vi "PH_PowerUnit_BaseClass.handle TO.vi"(0 "VI in":refnum<vi>, 2 "String":string, 5 "error in (no error)":errorcluster) -> (14 "VI out":refnum<vi>, 19 "error out":errorcluster)   [LabVIEW 2014, in "PH_PowerUnit_BaseClass.lvlib"]
uses:
  PH_PowerUnit_BaseClass.lvlib
  PHELIX/PH_Sequencer/PH_Sequencer.lvlib
  PH_Common/PH_Common.lvlib
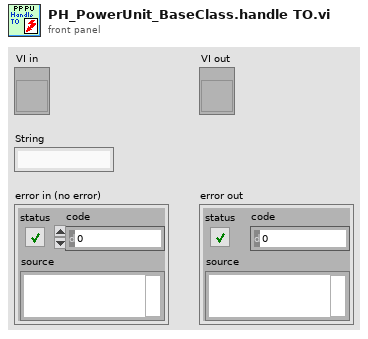
[diagram p1: front panel]
types:
  T1 = typedef "PH_PowerUnit_BaseClass.lvlib/PH_PowerUnit_BaseClass.i attribute.ctl" = cluster{"Constructor finished":bool, "PU":cluster{"In use":bool, "Service ID in use":i32, "GUI Ref":refnum<vi>}, "Enabling":cluster{"State":T2, "GUI Ref":refnum<vi>}, "Timing":cluster{"Last Shot":dbl, "Time between Shots [Sec]":dbl, "Waiting Time over?":bool, "Service ID Waiting Time":i32, "GUI Ref":refnum<vi>, "Instance":cluster{"Status":T3, "linked?":bool, "GUI Ref":refnum<vi>}}, "Sequencer":cluster{"SM State":string, "GUI Ref":refnum<vi>, "linked":bool}, "Subscribed Trendmssgs":cluster{"Tagname":string, "Status":T3, "linked?":bool, "Shot Condition":T3, "GUI Ref":refnum<vi>}[], "PP PU":T4, "Default Voltage (V)":dbl, "GUI Refs":T5, "PSDB data":cluster{"Shot Voltage [V]":dbl, "State TO SM":T6, "Write 2 early":bool}, "State TO SM":T6}
  T2 = typedef "PH_SystemInformation.lvlib/PH_SystemInformationEnabling State.ctl" = i32
  T3 = typedef "PH_StatusHandler.lvlib/PH_StatusHandler.Status.ctl" = i16
  T4 = typedef "PH_PP_Common.lvlib/PH_PP_Common.PUs.ctl" = enum16{"no Info", "PA-19mm-1", "PA-19mm-2", "PA-45mm-PILC", "PA-45mm-MAIN", "MA-PU-1", "MA-PU-2", "MA-PU-3", "MA-PU-4", "MA-PU-5", "MA-PU-6", "MA-FR", "MA-PILC", "PA-45mm-DP"}
  T5 = typedef "PH_PowerUnit_BaseClass.lvlib/PH_PowerUnit_BaseClass.GUI Refs.ctl" = cluster{"Delete Inst":refnum<vi>, "State TO SM":refnum<vi>, "State SM":refnum<vi>, "Fire":refnum<vi>}
  T6 = typedef "PH_PowerUnit_BaseClass.lvlib/PH_PowerUnit_BaseClass.SM States.ctl" = enum16{".", "Stand by", "Switch PU on", "Configure", "Set Default Voltage", "Set STANDBY", "Set READY", "Wait for Shot Cmd", "Open Dump Rods", "Open Ross Relais", "Close Ross Relais", "Switch PSU on", "Switch PSU off", "Charge", "Switch GD Channel on", "Close Dump Rods", "Rods-TO", "RR-TO", "PSU-TO", "Trigger-TO"}
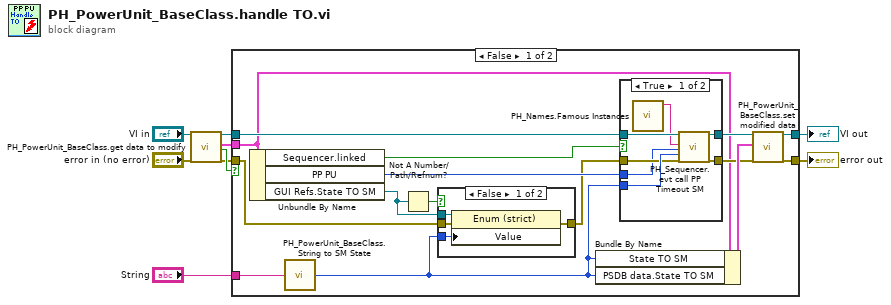
[diagram p0: block diagram]
diagram:
  n1 = call "PH_PowerUnit_BaseClass.get data to modify.vi"("i ref in"="VI in", "error in (no error)"="error in (no error)") -> ("i ref out"=w1:refnum<vi>, "i attribute"=w3:T1, "timed out"=w4:bool, "error out"=w2:errorcluster)  [unwired: 14 in]
  n2 = case shown="False" w4 {
    tunnel: w1 -> [w17 w40]
    tunnel: [w24 w40] -> w7
    tunnel: w2 -> [w21 w39]
    tunnel: [w23 w39] -> w8
    tunnel: w3 -> [w15 _]
    tunnel: "String" -> [w20 _]
    frame False {
      n3 = Unbundle By Name(w15) -> ("Sequencer.linked"=w14:bool, "PP PU"=w18:T4, "GUI Refs.State TO SM"=w10:refnum<vi>)
      n4 = call "PH_PowerUnit_BaseClass.String to SM State.vi"("SM State String"=w20) -> ("SM State"=w13:T6)
      n5 = Not A Number/Path/Refnum?(number/path/refnum=w10) -> (NaN/Path/Refnum?=w11:bool)
      n6 = case shown="False" w11 {
        tunnel: w21 -> [w28 w29]
        tunnel: w10 -> [w27 _]
        tunnel: w13 -> [w26 _]
        tunnel: [w25 w29] -> w12
        frame False {
          n7 = property class="Enum (strict)"(reference=w27, error in=w28, "Value"=w26) -> (error out=w25:errorcluster)  [unwired: 1 out]
        }
        frame True {
        }
      }
      n8 = Bundle By Name(cluster=w15, "State TO SM"=w13, "PSDB data.State TO SM"=w13) -> (w22:T1)
      n9 = case shown="True" w14 {
        tunnel: w17 -> [w32 w38]
        tunnel: [w36 w38] -> w16
        tunnel: w12 -> [w33 w37]
        tunnel: [w35 w37] -> w19
        tunnel: w13 -> [w34 _]
        tunnel: w18 -> [w31 _]
        frame True {
          n10 = call "PH_Names.Famous Instances.vi"() -> ("Sequencer"=w30:string)  [unwired: 7 in, 3 out]
          n11 = call "PH_Sequencer.evt call PP Timeout SM.vi"("i ref in"=w32, "Instance"=w30, "Power Unit"=w31, "PP Timeout SM"=w34, "error in (no error)"=w33) -> ("i ref out"=w36:refnum<vi>, "error out"=w35:errorcluster)  [unwired: 13 in]
        }
        frame False {
        }
      }
      n12 = call "PH_PowerUnit_BaseClass.set modified data.vi"("i ref in"=w16, "i attribute"=w22, "error in (no error)"=w19) -> ("i ref out"=w24:refnum<vi>, "error out"=w23:errorcluster)  [unwired: 15 in]
    }
    frame True {
    }
  }
  "error out" <- w8
  "VI out" <- w7
